vi "获取最近两组水样测试数据.vi"(8 "error in (no error)":errorcluster, 11 "table":string) -> (0 "error out":errorcluster, 3 "存储变量":T1)   [LabVIEW 2016, in "PLC.lvlib"]
uses:
  PLC.lvlib
  <vilib>/Utility/sysdir.llb/System Directory Type.ctl
  <vilib>/addons/database/Connection.llb/DB Tools Open Connec (String).vi
  <vilib>/addons/database/Connection.llb/Conn Execute.vi
  <vilib>/addons/database/Recordset.llb/Rec Fetch Recordset Data (R).vi
  <vilib>/addons/database/Recordset.llb/Rec Destroy - Connection.vi
  <vilib>/addons/database/_DB Variant To Data/Database Variant To Data.xnode
  <vilib>/addons/database/NI_Database_API.lvlib
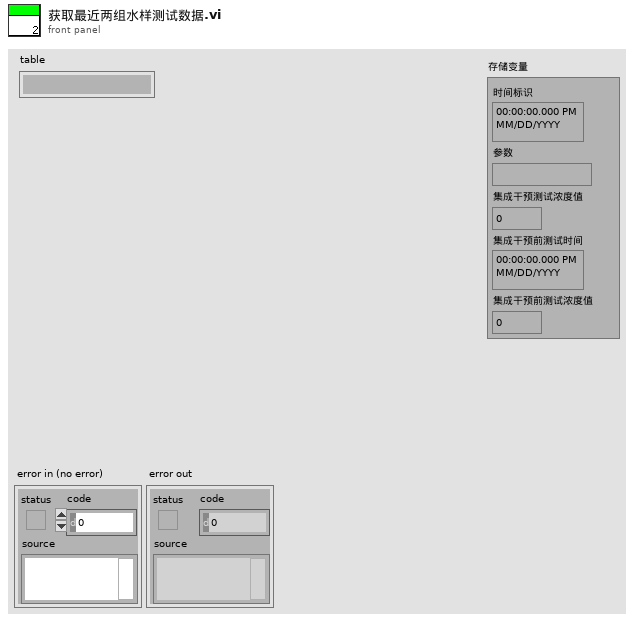
[diagram p1: front panel]
types:
  T1 = cluster{"时间标识":timestamp, "参数":string, "集成干预测试浓度值":dbl, "集成干预前测试时间":timestamp, "集成干预前测试浓度值":dbl}
  T2 = typedef "System Directory Type.ctl" = i32
  T3 = typedef "NI_Database_API.lvlib/Conn ObjectReference.ctl" = refnum<k1>
  T4 = typedef "NI_Database_API.lvlib/Rec ObjectReference.ctl" = refnum<k1>
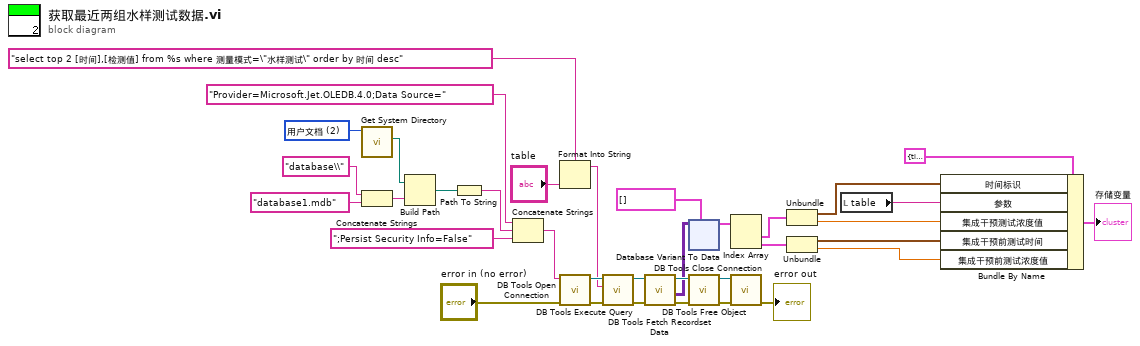
[diagram p0: block diagram]
diagram:
  w33 = T2 2 items=["用户目录"=0, "用户桌面"=1, "用户文档"=2, "用户应用程序数据"=3, "用户设置"=4, "用户临时目录"=5, "公共文档"=6, "公共应用程序数据"=7, "公共设置"=8, "公共缓存"=13, "系统核心库"=9, "系统安装库"=10, "应用程序文件"=11, "启动盘根目录"=12] ("system directory type")
  n1 = call <vilib>:"Get System Directory.vi"("system directory type"=w33) -> ("system directory"=w31:path)  [unwired: 10 in]
  n2 = Concatenate Strings("database\\" ("condition"), "database1.mdb" ("condition")) -> (w25:string)
  n3 = Build Path(base path=w31, name or relative path=w25) -> (appended path=w30:path)
  n4 = Path To String(path=w30) -> (string=w29:string)
  n5 = Concatenate Strings("Provider=Microsoft.Jet.OLEDB.4.0;Data Source=" ("condition"), w29, ";Persist Security Info=False" ("condition")) -> (w27:string)
  n6 = Format Into String(format string="select top 2 [时间],[检测值] from %s where 测量模式=\"水样测试\" order by 时间 desc" ("格式字符串"), "table") -> (resulting string=w14:string)  [unwired: 2 in, 1 out]
  n7 = call-poly <vilib>:"DB Tools Open Connection.vi"("error in (no error)"="error in (no error)", "connection information"=w27) -> ("error out"=w20:errorcluster, "connection reference"=w21:T3)  [unwired: 6 in]
  n8 = call-poly <vilib>:"DB Tools Execute Query.vi"("error in (no error)"=w20, "SQL query"=w14, "connection reference"=w21) -> ("error out"=w19:errorcluster, "recordset reference"=w24:T4)  [unwired: 5 in]
  n9 = call-poly <vilib>:"DB Tools Fetch Recordset Data.vi"("error in (no error)"=w19, "recordset reference"=w24) -> ("error out"=w22:errorcluster, "recordset data"=w12:variant[][], "recordset reference out"=w23:T4)  [unwired: 3 in]
  n10 = xnode "Database Variant To Data"("database variant"=w12, "type"=cluster{"时间":timestamp, "检测值 ":dbl}[] []) -> ("data"=w9:cluster{timestamp, dbl}[])  [unwired: 1 in, 1 out]
  n11 = call-poly <vilib>:"DB Tools Free Object.vi"("error in (no error)"=w22, "recordset reference"=w23) -> ("error out"=w17:errorcluster, "connection reference"=w18:T3)  [unwired: 8 in]
  n12 = Index Array(array=w9) -> (element #1=w8:cluster{timestamp, dbl}, element #2=w5:cluster{timestamp, dbl})  [unwired: 2 in]
  n13 = call <vilib>:"DB Tools Close Connection.vi"("error in (no error)"=w17, "connection reference"=w18) -> ("error out"=→"error out":errorcluster)  [unwired: 5 in]
  n14 = Unbundle(w8) -> (w7:timestamp, w6:dbl)
  n15 = Unbundle(w5) -> (w4:timestamp, w3:dbl)
  n16 = local read "table"() -> (w10:string)
  n17 = Bundle By Name(cluster=T1 {"时间标识"=timestamp(0 s since 1904-01-01), "参数"="", "集成干预测试浓度值"=0.0, "集成干预前测试时间"=timestamp(0 s since 1904-01-01), "集成干预前测试浓度值"=0.0} ("存储变量"), "时间标识"=w7, "参数"=w10, "集成干预测试浓度值"=w6, "集成干预前测试时间"=w4, "集成干预前测试浓度值"=w3) -> (→"存储变量":T1)
